vi "Switch Configuration - Filter Topologies by Switch Model.vi"(8 "error in (no error)":errorcluster, 11 "Switch Config UI Data In":T1 {"Switch Config Page Item Ref" format="%.0x"}) -> (0 "error out":errorcluster, 2 "First Topology from List":string, 3 "Switch Config UI Data Out":T1 {"Switch Config Page Item Ref" format="%.0x"})   [LabVIEW 2015, in "DMM-SWITCH-ScanList System Explorer.lvlib"]
doc: "Update the Topology Control with the supported topologies for a specific switch model."
uses:
  DMM-SWITCH-ScanList System Explorer.lvlib
  Configuration Controls/Switch Config VI UI Data.ctl
  Configuration Controls/Switch Config VI UI Ctrl Values.ctl
  Configuration Controls/Switch Config VI UI Ctrl References.ctl
  <instrlib>/niSwitch/niSwitch.LLB/niSwitch Topologies.ctl
  <vilib>/NI Veristand/Custom Device API/Custom Device Item Ref.ctl
  <vilib>/NI Veristand/Custom Device API/Custom Device API.lvlib
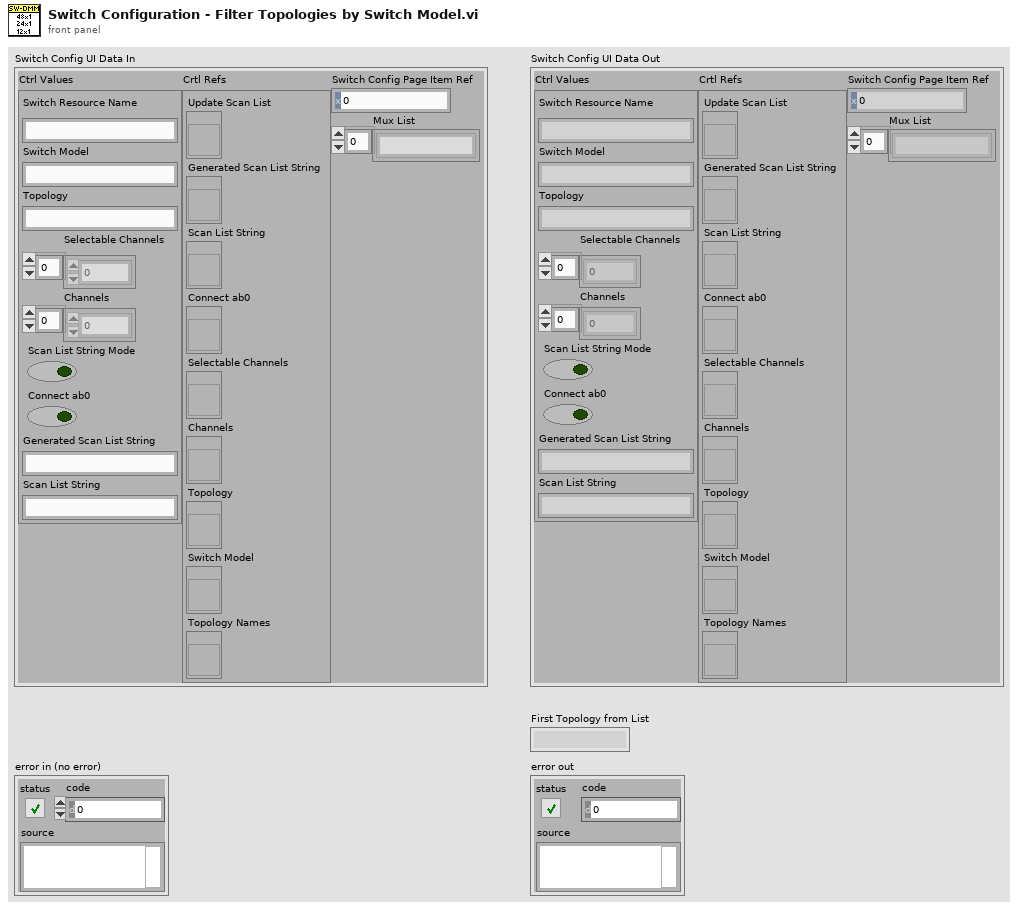
[diagram p1: front panel]
types:
  T1 = typedef "DMM-SWITCH-ScanList System Explorer.lvlib/Switch Config VI UI Data.ctl" = cluster{"Ctrl Values":T2, "Crtl Refs":T3, "Switch Config Page Item Ref":T4, "Mux List":string[]}
  T2 = typedef "DMM-SWITCH-ScanList System Explorer.lvlib/Switch Config VI UI Ctrl Values.ctl" = cluster{"Switch Resource Name":string, "Switch Model":string, "Topology":string, "Selectable Channels":i32[], "Channels":i32[], "Scan List String Mode":bool, "Connect ab0":bool, "Generated Scan List String":string, "Scan List String":string}
  T3 = typedef "DMM-SWITCH-ScanList System Explorer.lvlib/Switch Config VI UI Ctrl References.ctl" = cluster{"Update Scan List":refnum<vi>, "Generated Scan List String":refnum<vi>, "Scan List String":refnum<vi>, "Connect ab0":refnum<vi>, "Selectable Channels":refnum<vi>, "Channels":refnum<vi>, "Topology":refnum<vi>, "Switch Model":refnum<vi>, "Topology Names":refnum<vi>}
  T4 = typedef "Custom Device API.lvlib/Custom Device Item Ref.ctl" = u64
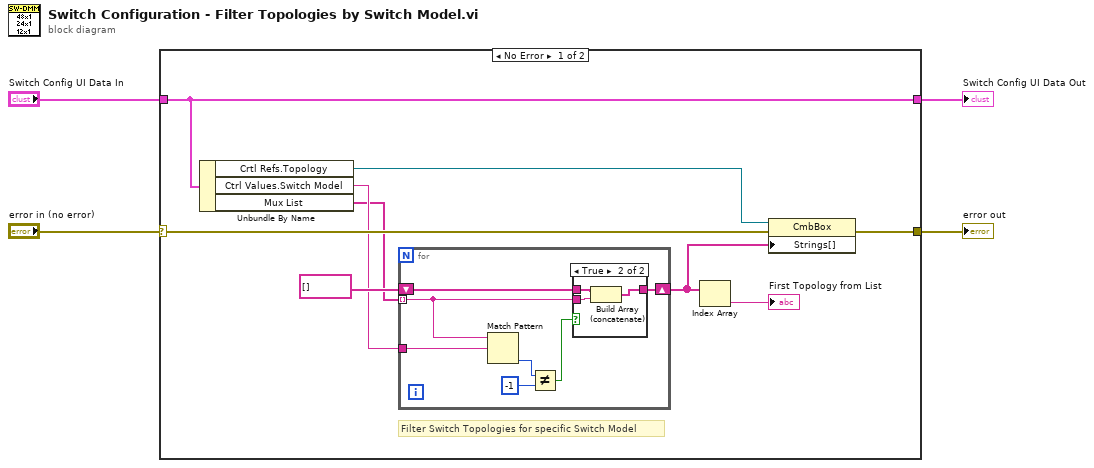
[diagram p0: block diagram]
diagram:
  n1 = case shown="No Error" "error in (no error)" {
    selector: "error in (no error)" -> [w9 w26]
    tunnel: [w10 w26] -> w4
    tunnel: "Switch Config UI Data In" -> [w5 w25]
    tunnel: [w5 w25] -> w1
    frame No Error {
      # "Filter Switch Topologies for specific Switch Model"
      n2 = Unbundle By Name(w5) -> ("Crtl Refs.Topology"=w8:refnum<vi>, "Ctrl Values.Switch Model"=w7:string, "Mux List"=w6:string[])
      n3 = for {
        tunnel: w6 -> [w16] mode=indexing
        tunnel: w7 -> [w17]
        shift-right: [w14] -> w13
        shift-left: string[] [] ("Strings []") -> [w15]
        n4 = Match Pattern(string=w16, regular expression=w17) -> (offset past match=w19:i32)  [unwired: 1 in, 3 out]
        n5 = Not Equal?(x=w19, y=-1) -> (x != y?=w20:bool)
        n6 = case shown="True" w20 {
          tunnel: w15 -> [w21 w24]
          tunnel: w16 -> [_ w23]
          tunnel: [w21 w22] -> w14
          frame False {
          }
          frame True {
            n7 = Build Array (concatenate)(w24, w23) -> (w22:string[])
          }
        }
      }
      n8 = Index Array(array=w13) -> (element=→"First Topology from List":string)  [unwired: 1 in]
      n9 = property on="Property Node" class="CmbBox"(reference=w8, error in=w9, "Strings[]"=w13) -> (error out=w10:errorcluster)  [unwired: 1 out]
    }
    frame Error {
    }
  }
  "error out" <- w4
  "Switch Config UI Data Out" <- w1
